vi "Set enable state on multiple controle.vi"(9 "Booléen":bool, 11 "Ref. Tab":refnum<vi>[](array[refnum])) -> ()   [LabVIEW 2017, in "IHM Control.lvlib"]
uses:
  IHM Control.lvlib
panel:
  out "Tableau":errorcluster[](array[cluster])
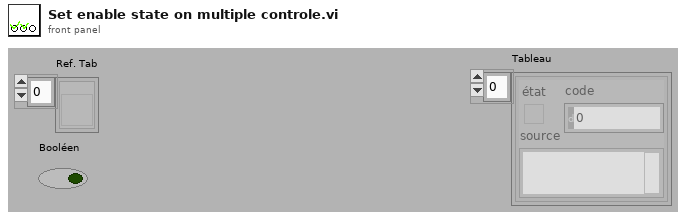
[diagram p1: front panel]
types:
  T1 = enum8{"Enabled", "Disabled", "Disabled and Grayed Out"}
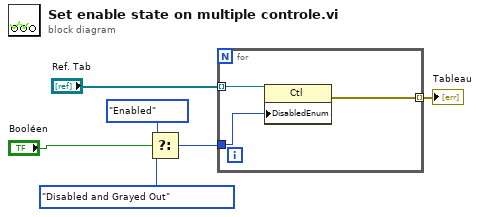
[diagram p0: block diagram]
diagram:
  n1 = Select(t=T1."Enabled" ("Désactivé"), s="Booléen", f=T1."Disabled and Grayed Out" ("Désactivé")) -> (s? t:f=w2:T1)
  n2 = for {
    tunnel: "Ref. Tab" -> [w9] mode=indexing
    tunnel: w2 -> [w8]
    tunnel: [w7] -> w1 mode=indexing
    n3 = property class="Ctl"(reference=w9, "DisabledEnum"=w8) -> (error out=w7:errorcluster)  [unwired: 1 in, 1 out]
  }
  "Tableau" <- w1
